vi "Test read value.vi"() -> ()   [LabVIEW 2017]
panel:
  out "current time 2":timestamp
  out "current time":timestamp
  out "Distance OUT2":dbl[](array[numeric])
  out "Measurement time, ms 2":dbl[](array[numeric])
  in  "stop":bool
  out "Measurement time, ms":dbl[](array[numeric])
  out "Distance OUT1":dbl[](array[numeric])
  in  "Rate":enum16{"9600", "115200"}(ring)=enum."115200"
  in  "VISA resource name":refnum<visa-resource-name>="COM1"
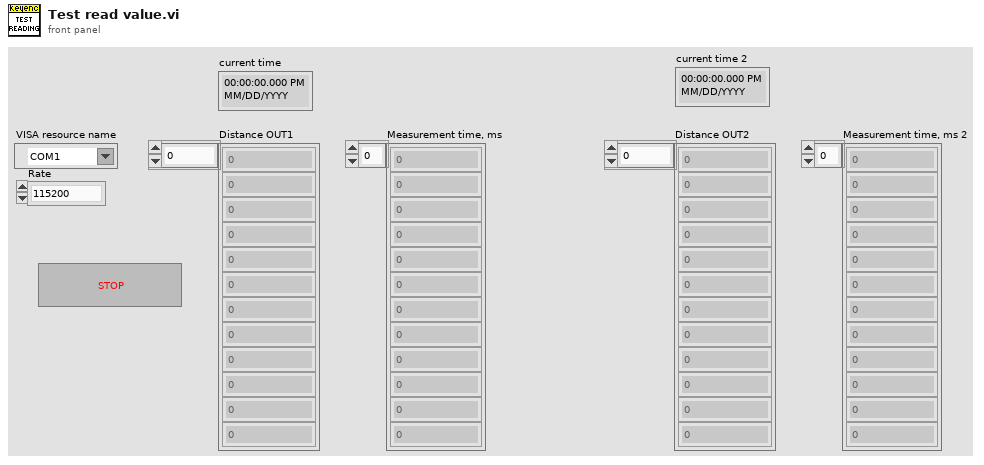
[diagram p1: front panel]
types:
  T1 = typedef "Semaphore RefNum" = refnum<k1>
  T2 = cluster{"Serial port sem":T1, "Serial port handle":refnum<visa-resource-name>, "Baud rate":u32}
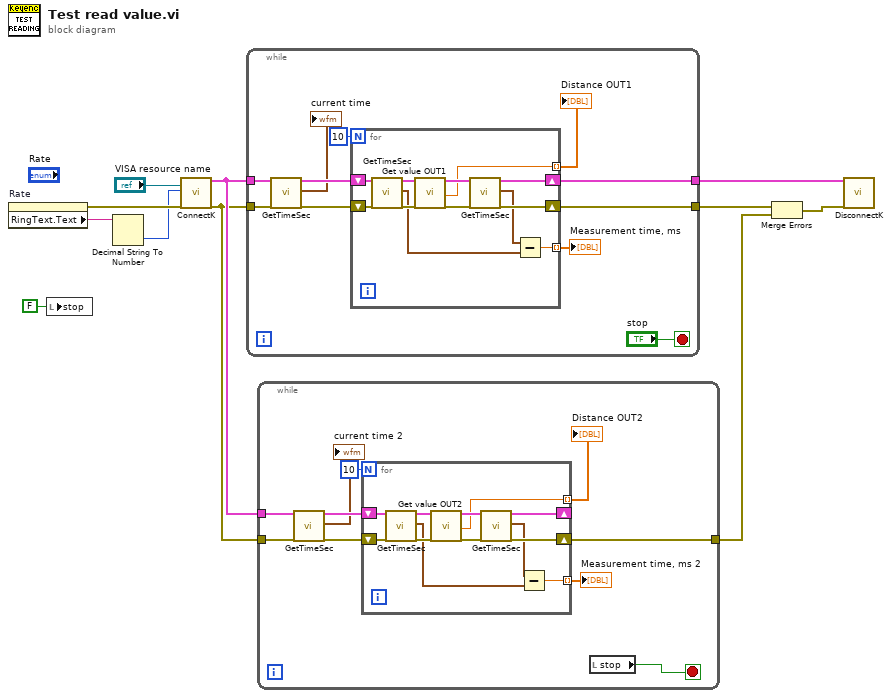
[diagram p0: block diagram]
diagram:
  n1 = property on="Rate" class="Enum (strict)"() -> (error out=w11:errorcluster, "RingText.Text"=w10:string)  [unwired: 2 in, 1 out]
  n2 = local write "stop"(FALSE ("stop")) -> ()
  n3 = Decimal String To Number(string=w10) -> (number=w9:i32)  [unwired: 2 in, 1 out]
  n4 = call "ConnectK.vi"("VISA resource name"="VISA resource name", "Baud rate"=w9, "error in"=w11) -> ("Keyence"=w7:T2, "error out"=w2:errorcluster)  [unwired: 15 in]
  n5 = while {
    tunnel: w7 -> [w21]
    tunnel: [w20] -> w1
    tunnel: w2 -> [w14]
    tunnel: [w18] -> w5
    stop <- "stop" stop-if-true
    n6 = call "GetTimeSec.vi"("error in"=w14) -> ("current time"=→"current time":timestamp, "error out"=w13:errorcluster)  [unwired: 17 in]
    n7 = for {
      N: 10 -> [_]
      tunnel: [w22] -> w19 mode=indexing
      tunnel: [w25] -> w16 mode=indexing
      shift-right: [w27] -> w18
      shift-left: w13 -> [w30]
      shift-right: [w31] -> w20
      shift-left: w21 -> [w23]
      n8 = call "GetTimeSec.vi"("error in"=w30) -> ("current time"=w26:timestamp, "error out"=w29:errorcluster)  [unwired: 17 in]
      n9 = call "Get value OUT1.vi"("Keyence"=w23, "error in"=w29) -> ("Keyence out"=w31:T2, "Distance"=w22:dbl, "error out"=w28:errorcluster)  [unwired: 14 in, 1 out]
      n10 = call "GetTimeSec.vi"("error in"=w28) -> ("current time"=w24:timestamp, "error out"=w27:errorcluster)  [unwired: 17 in]
      n11 = Subtract(x=w24, y=w26) -> (x-y=w25:dbl)
    }
    "Distance OUT1" <- w19
    "Measurement time, ms" <- w16
  }
  n12 = while {
    tunnel: w7 -> [w40]
    tunnel: w2 -> [w34]
    tunnel: [w38] -> w4
    stop <- w35 stop-if-true
    n13 = call "GetTimeSec.vi"("error in"=w34) -> ("current time"=→"current time 2":timestamp, "error out"=w33:errorcluster)  [unwired: 17 in]
    n14 = for {
      N: 10 -> [_]
      tunnel: [w41] -> w39 mode=indexing
      tunnel: [w44] -> w36 mode=indexing
      shift-right: [w46] -> w38
      shift-left: w33 -> [w49]
      shift-right: [w50] -> _
      shift-left: w40 -> [w42]
      n15 = call "GetTimeSec.vi"("error in"=w49) -> ("current time"=w45:timestamp, "error out"=w48:errorcluster)  [unwired: 17 in]
      n16 = call "Get value OUT2.vi"("Keyence"=w42, "error in"=w48) -> ("Keyence out"=w50:T2, "Distance"=w41:dbl, "error out"=w47:errorcluster)  [unwired: 13 in, 2 out]
      n17 = call "GetTimeSec.vi"("error in"=w47) -> ("current time"=w43:timestamp, "error out"=w46:errorcluster)  [unwired: 17 in]
      n18 = Subtract(x=w43, y=w45) -> (x-y=w44:dbl)
    }
    "Distance OUT2" <- w39
    "Measurement time, ms 2" <- w36
    n19 = local read "stop"() -> (w35:bool)
  }
  n20 = Merge Errors(w5, w4) -> (w3:errorcluster)
  n21 = call "DisconnectK.vi"("Keyence"=w1, "error in"=w3) -> ()  [unwired: 17 in, 1 out]
